vi "8-bit compatator.vi"(8 "q":enum16{"", "1", "0"}(ring), 11 "P":enum16{"", "1", "0"}(ring)) -> (0 "Czy p>q?":bool, 3 "Czy p=q?":bool)   [LabVIEW 2020]
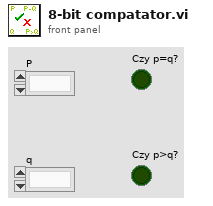
[diagram p1: front panel]
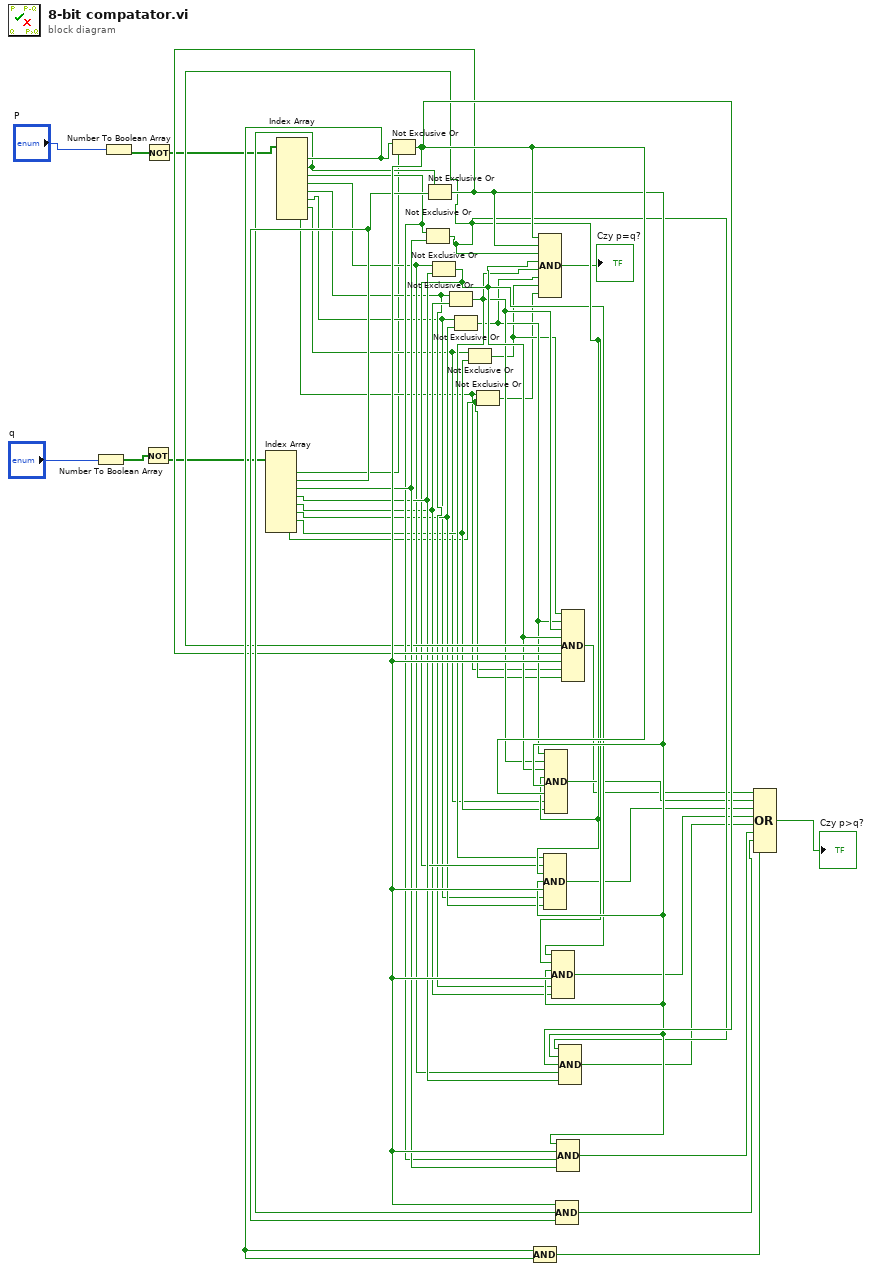
[diagram p0: block diagram]
diagram:
  n1 = Number To Boolean Array(number="q") -> (Boolean array=w1:bool[])
  n2 = Number To Boolean Array(number="P") -> (Boolean array=w3:bool[])
  n3 = Not(x=w1) -> (.not. x?=w2:bool[])
  n4 = Not(x=w3) -> (.not. x?=w4:bool[])
  n5 = Index Array(array=w2) -> (element #1=w5:bool, element #2=w38:bool, element #3=w32:bool, element #4=w28:bool, element #5=w23:bool, element #6=w20:bool, element #7=w16:bool, element #8=w13:bool)  [unwired: 8 in]
  n6 = Index Array(array=w4) -> (element #1=w40:bool, element #2=w37:bool, element #3=w31:bool, element #4=w27:bool, element #5=w22:bool, element #6=w19:bool, element #7=w15:bool, element #8=w12:bool)  [unwired: 8 in]
  n7 = Not Exclusive Or(1:w5, 2:w40) -> (0:w39:bool)
  n8 = Not Exclusive Or(1:w32, 2:w31) -> (0:w29:bool)
  n9 = Not Exclusive Or(1:w38, 2:w37) -> (0:w33:bool)
  n10 = Not Exclusive Or(1:w28, 2:w27) -> (0:w24:bool)
  n11 = Not Exclusive Or(1:w23, 2:w22) -> (0:w21:bool)
  n12 = Not Exclusive Or(1:w20, 2:w19) -> (0:w17:bool)
  n13 = Not Exclusive Or(1:w16, 2:w15) -> (0:w11:bool)
  n14 = Not Exclusive Or(1:w13, 2:w12) -> (0:w9:bool)
  n15 = Compound Arithmetic op=AND(w40, w40) -> (w36:bool)
  n16 = Compound Arithmetic op=AND(w39, w33, w29, w24, w21, w17, w11, w9) -> (→"Czy p=q?":bool)
  n17 = Compound Arithmetic op=AND(w21, w24, w29, w33, w39, w19, w20) -> (w18:bool)
  n18 = Compound Arithmetic op=AND(w17, w21, w24, w29, w33, w39, w15, w16) -> (w14:bool)
  n19 = Compound Arithmetic op=AND(w24, w29, w33, w39, w22, w23) -> (w25:bool)
  n20 = Compound Arithmetic op=AND(w39, w37, w38) -> (w35:bool)
  n21 = Compound Arithmetic op=AND(w33, w39, w31, w32) -> (w30:bool)
  n22 = Compound Arithmetic op=AND(w29, w33, w39, w27, w28) -> (w26:bool)
  n23 = Compound Arithmetic op=AND(w11, w17, w21, w24, w29, w33, w39, w12, w13) -> (w10:bool)
  n24 = Compound Arithmetic op=OR(w10, w14, w18, w25, w26, w30, w35, w36) -> (→"Czy p>q?":bool)
